vi "Motor_generatemotion.vi"(1 "Conversion\n (steps/mm)":dbl[](array[numeric])=[12500.0, 31496.063, 31496.063, 31496.063] format="%#_13g", 2 "Distance  (mm)":dbl[](array[numeric])=[0.0, 0.0, 0.0, 0.0] format="%#_13g") -> (0 "Movement string":string)   [LabVIEW 2015]
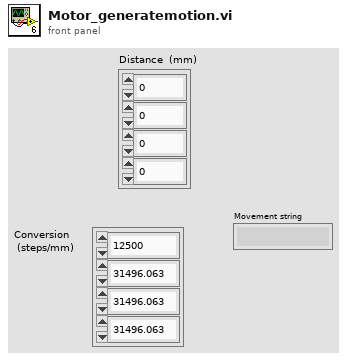
[diagram p1: front panel]
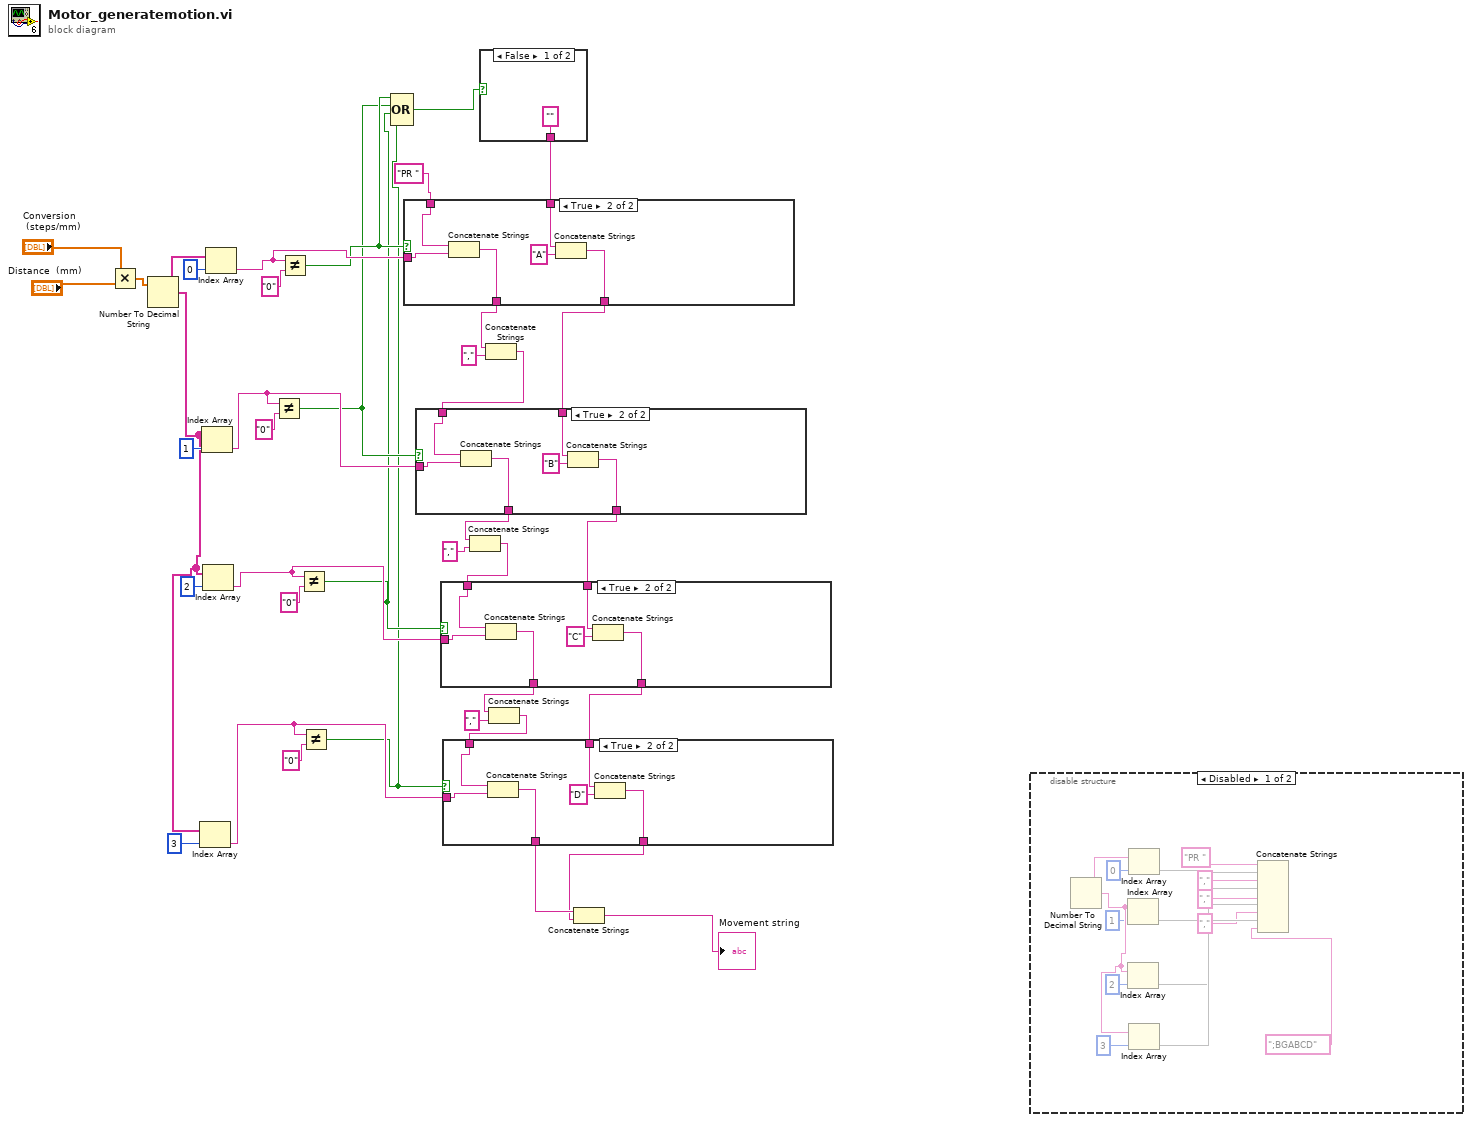
[diagram p0: block diagram]
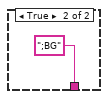
[diagram p2: hidden frame]
diagram:
  n1 = Multiply(x="Conversion\n (steps/mm)", y="Distance  (mm)") -> (x*y=w38:dbl[])
  n2 = Number To Decimal String(number=w38) -> (decimal integer string=w31:string[])  [unwired: 1 in]
  n3 = Index Array(array=w31, index=3) -> (element=w21:string)
  n4 = Index Array(array=w31, index=1) -> (element=w26:string)
  n5 = Index Array(array=w31, index=2) -> (element=w23:string)
  n6 = Index Array(array=w31, index=0) -> (element=w28:string)
  n7 = Not Equal?(x=w26, y="0") -> (x != y?=w5:bool)
  n8 = Not Equal?(x=w28, y="0") -> (x != y?=w6:bool)
  n9 = Not Equal?(x=w23, y="0") -> (x != y?=w4:bool)
  n10 = Not Equal?(x=w21, y="0") -> (x != y?=w3:bool)
  n11 = Compound Arithmetic op=OR(w6, w5, w4, w3) -> (w1:bool)
  n12 = case shown="False" w1 {
    tunnel: ["" ("string") ";BG" ("string")] -> w2
    frame False {
    }
    frame True {
    }
  }
  n13 = case shown="True" w6 {
    tunnel: "PR " ("string") -> [w42 w48]
    tunnel: w2 -> [w41 w46]
    tunnel: w28 -> [_ w47]
    tunnel: [w41 w44] -> w13
    tunnel: [w42 w43] -> w16
    frame False {
    }
    frame True {
      n14 = Concatenate Strings(w48, w47) -> (w43:string)
      n15 = Concatenate Strings(w46, "A" ("string")) -> (w44:string)
    }
  }
  n16 = Concatenate Strings(w16, "," ("string")) -> (w14:string)
  n17 = case shown="True" w5 {
    tunnel: w14 -> [w50 w56]
    tunnel: w13 -> [w49 w54]
    tunnel: w26 -> [_ w55]
    tunnel: [w49 w52] -> w24
    tunnel: [w50 w51] -> w12
    frame False {
    }
    frame True {
      n18 = Concatenate Strings(w56, w55) -> (w51:string)
      n19 = Concatenate Strings(w54, "B" ("string")) -> (w52:string)
    }
  }
  n20 = Concatenate Strings(w12, "," ("string")) -> (w7:string)
  n21 = case shown="True" w4 {
    tunnel: w7 -> [w58 w64]
    tunnel: w24 -> [w57 w62]
    tunnel: w23 -> [_ w63]
    tunnel: [w57 w60] -> w20
    tunnel: [w58 w59] -> w9
    frame False {
    }
    frame True {
      n22 = Concatenate Strings(w64, w63) -> (w59:string)
      n23 = Concatenate Strings(w62, "C" ("string")) -> (w60:string)
    }
  }
  n24 = Concatenate Strings(w9, "," ("string")) -> (w8:string)
  n25 = case shown="True" w3 {
    tunnel: w8 -> [w66 w72]
    tunnel: w20 -> [w65 w70]
    tunnel: w21 -> [_ w71]
    tunnel: [w65 w68] -> w18
    tunnel: [w66 w67] -> w19
    frame False {
    }
    frame True {
      n26 = Concatenate Strings(w72, w71) -> (w67:string)
      n27 = Concatenate Strings(w70, "D" ("string")) -> (w68:string)
    }
  }
  n28 = Concatenate Strings(w19, w18) -> (→"Movement string":string)
  n29 = disable-structure shown="Disabled" {
    frame Disabled {
      n30 = Number To Decimal String() -> (decimal integer string=w84:string)  [unwired: 2 in]
      n31 = Index Array(array=w84, index=1) -> (element=w78)
      n32 = Index Array(array=w84, index=2) -> (element=w81)
      n33 = Index Array(array=w84, index=0) -> (element=w76)
      n34 = Index Array(array=w84, index=3) -> (element=w87)
      n35 = Concatenate Strings("PR " ("string"), w76, "," ("string"), w78, "," ("string"), w81, "," ("string"), w87, ";BGABCD" ("string")) -> (w82:string)
    }
    frame Enabled {
    }
  }
